vi "log_key_variant.vi"(8 "error in (no error)":errorcluster, 10 "Ctl Refnum":refnum<vi>, 11 "Byte Stream File in":refnum<file>) -> (0 "error out":errorcluster, 3 "Byte Stream File out":refnum<file>)   [LabVIEW 2015]
doc: "Copyright (c) 2018 Frans Korhonen, Institute for Atmospheric and Earth System Research / Physics, Faculty of Science, University of Helsinki, Finland\n\nThis file is part of MeasGUI.\n\nThis Source Code Form is subject to the terms of the Mozilla Public\nLicense, v. 2.0. If a copy of the MPL was not distributed with this\n file, You can obtain one at http://mozilla.org/MPL/2.0/."
panel:
  out "Value":variant
  out "ClassName":string
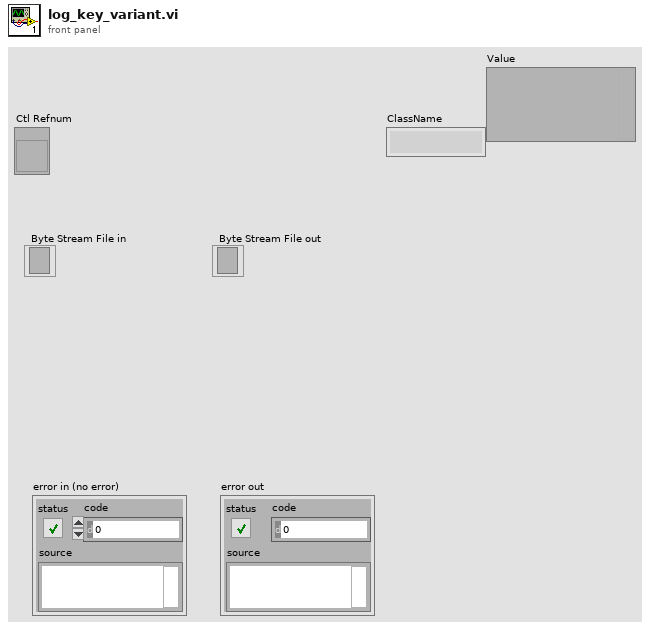
[diagram p1: front panel]
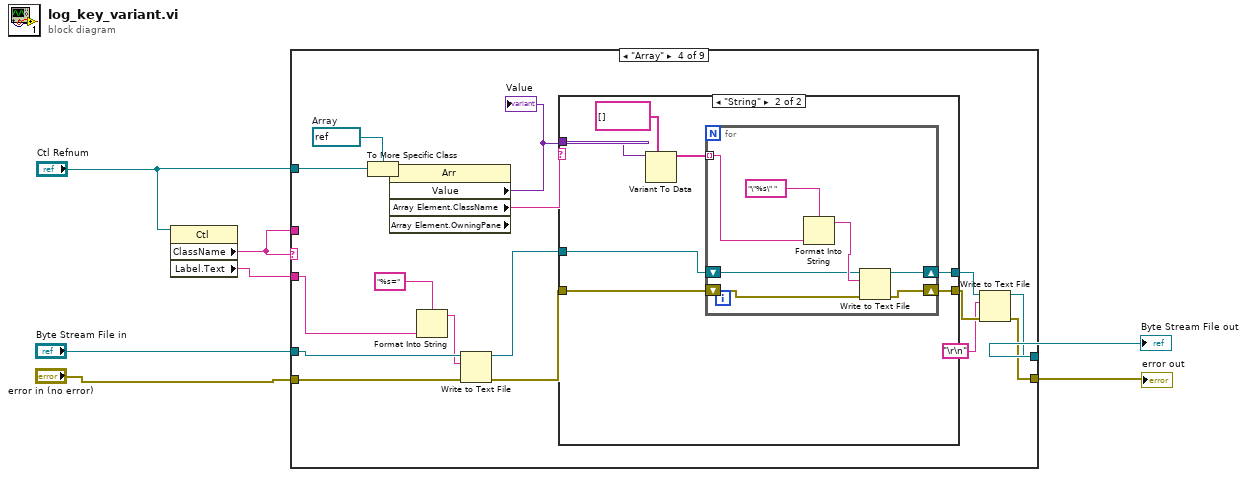
[diagram p0: block diagram]
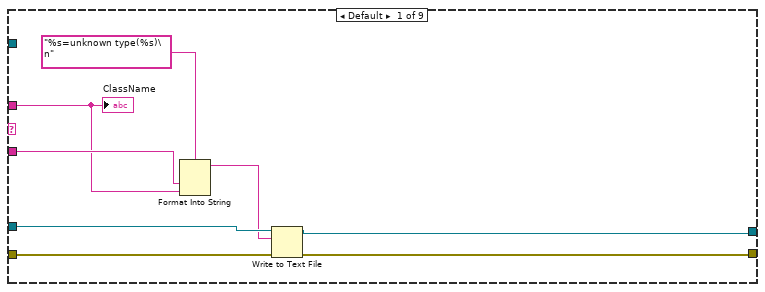
[diagram p2: hidden frame]
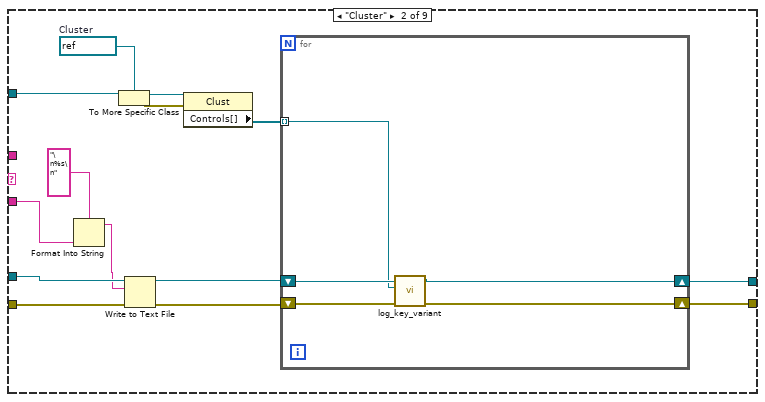
[diagram p3: hidden frame]
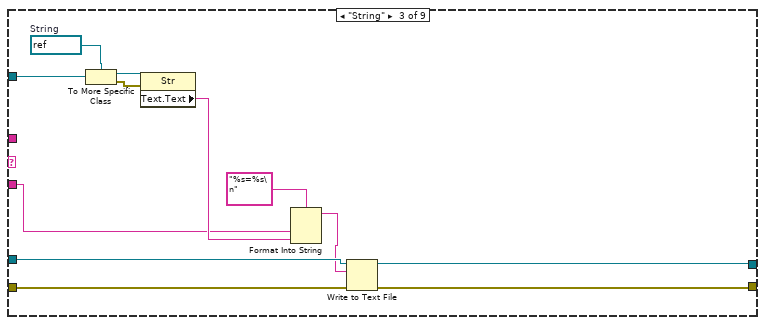
[diagram p4: hidden frame]
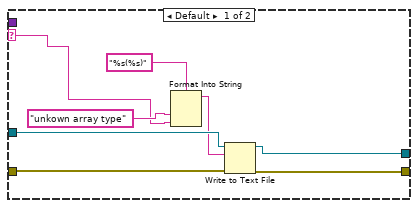
[diagram p5: hidden frame]
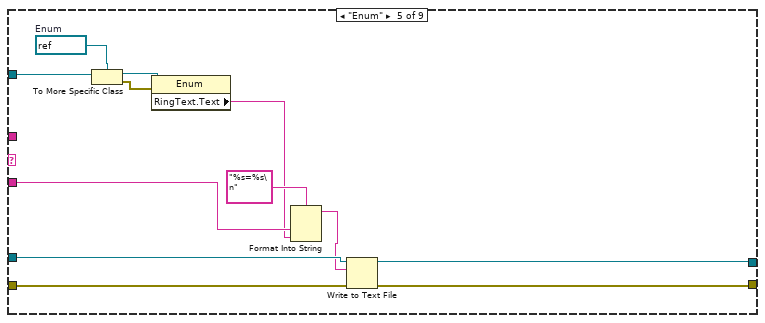
[diagram p6: hidden frame]
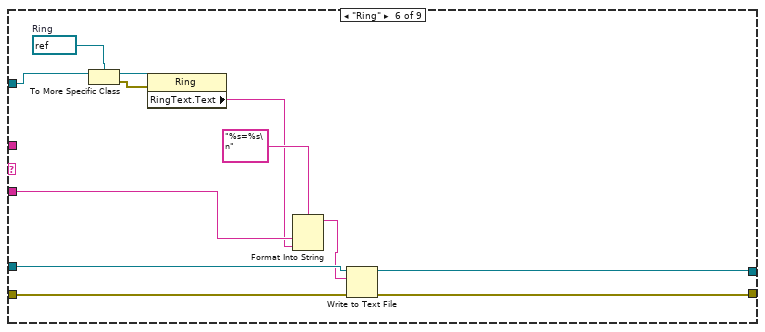
[diagram p7: hidden frame]
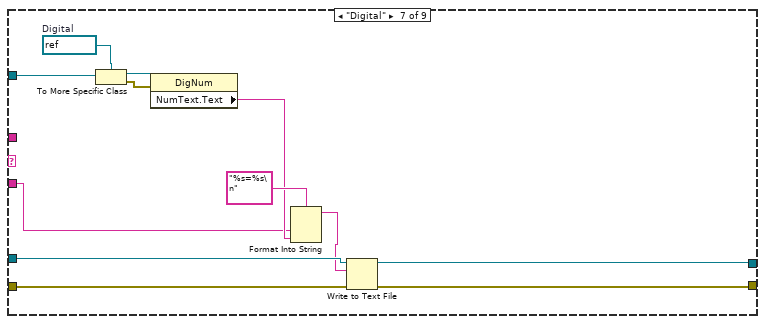
[diagram p8: hidden frame]
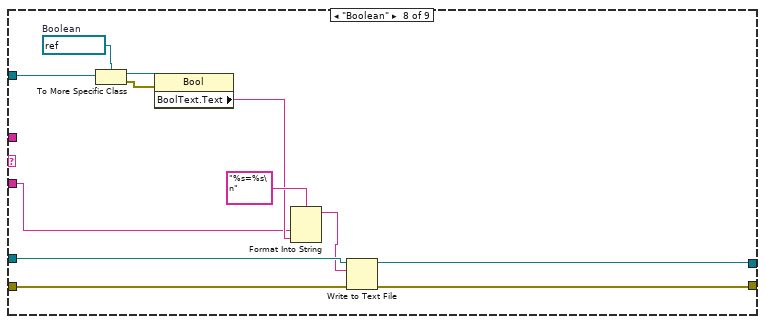
[diagram p9: hidden frame]
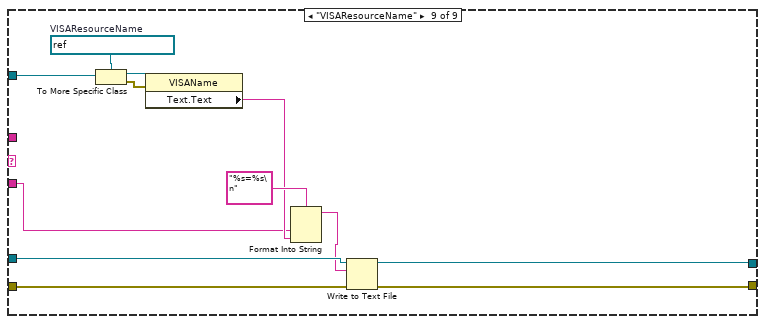
[diagram p10: hidden frame]
diagram:
  n1 = property class="Ctl"(reference="Ctl Refnum") -> ("ClassName"=w7:string, "Label.Text"=w1:string)  [unwired: 1 in, 2 out]
  n2 = case shown="\"Array\"" w7 {
    tunnel: w7 -> [w14 _ _ _ _ _ _ _ _]
    tunnel: "Ctl Refnum" -> [_ w28 w37 w61 w89 w101 w113 w125 w137]
    tunnel: "Byte Stream File in" -> [w12 w24 w46 w50 w98 w110 w122 w134 w146]
    tunnel: "error in (no error)" -> [w11 w23 w43 w51 w95 w107 w119 w131 w143]
    tunnel: [w10 w21 w45 w55 w97 w109 w121 w133 w145] -> w3
    tunnel: [w9 w18 w44 w56 w96 w108 w120 w132 w144] -> w2
    tunnel: w1 -> [w15 w17 w35 w47 w88 w100 w111 w123 w135]
    frame Default {
      n3 = Format Into String(format string="%s=unknown type(%s)\n", w15, w14) -> (resulting string=w8:string)  [unwired: 2 in, 1 out]
      n4 = Write to Text File(file (use dialog)=w12, text=w8, error in=w11) -> (refnum out=w10:refnum<file>, error out=w9:errorcluster)  [unwired: 1 in, 1 out]
      "ClassName" <- w14
    }
    frame "Cluster" {
      w29 = refnum<vi> refnum  # Cluster
      n5 = Format Into String(format string="\n%s\n", w17) -> (resulting string=w16:string)  [unwired: 2 in, 1 out]
      n6 = To More Specific Class(target class=w29, reference=w28) -> (specific class reference=w27:refnum<vi>, error out=w26:errorcluster)  [unwired: 1 in]
      n7 = Write to Text File(file (use dialog)=w24, text=w16, error in=w23) -> (refnum out=w20:refnum<file>, error out=w19:errorcluster)  [unwired: 1 in, 1 out]
      n8 = property class="Clust"(reference=w27, error in=w26) -> ("Controls[]"=w25:refnum<vi>[])  [unwired: 2 out]
      n9 = for {
        tunnel: w25 -> [w30] mode=indexing
        shift-right: [w34] -> w21
        shift-left: w20 -> [w33]
        shift-right: [w31] -> w18
        shift-left: w19 -> [w32]
        n10 = call "log_key_variant.vi"("error in (no error)"=w32, "Ctl Refnum"=w30, "Byte Stream File in"=w33) -> ("error out"=w31:errorcluster, "Byte Stream File out"=w34:refnum<file>)  [unwired: 7 in]
      }
    }
    frame "String" {
      w40 = refnum<vi> refnum  # String
      n11 = To More Specific Class(target class=w40, reference=w37) -> (specific class reference=w38:refnum<vi>, error out=w39:errorcluster)  [unwired: 1 in]
      n12 = property class="Str"(reference=w38, error in=w39) -> ("Text.Text"=w36:string)  [unwired: 2 out]
      n13 = Format Into String(format string="%s=%s\n", w35, w36) -> (resulting string=w42:string)  [unwired: 2 in, 1 out]
      n14 = Write to Text File(file (use dialog)=w46, text=w42, error in=w43) -> (refnum out=w45:refnum<file>, error out=w44:errorcluster)  [unwired: 1 in, 1 out]
    }
    frame "Array" {
      w64 = refnum<vi> refnum  # Array
      n15 = To More Specific Class(target class=w64, reference=w61) -> (specific class reference=w62:refnum<vi>, error out=w63:errorcluster)  [unwired: 1 in]
      n16 = property class="Arr" props=["Value", "Array Element", "ClassName", "Array Element", "OwningPane"](reference=w62, error in=w63) -> ("Value"=w60:variant, "Array Element.ClassName"=w59:string)  [unwired: 3 out]
      "Value" <- w60
      n17 = Format Into String(format string="%s=", w47) -> (resulting string=w49:string)  [unwired: 2 in, 1 out]
      n18 = Write to Text File(file (use dialog)=w50, text=w49, error in=w51) -> (refnum out=w53:refnum<file>, error out=w52:errorcluster)  [unwired: 1 in, 1 out]
      n19 = case shown="\"String\"" w59 {
        selector: w59 -> [w65 _]
        tunnel: w60 -> [_ w79]
        tunnel: w53 -> [w70 w76]
        tunnel: w52 -> [w69 w75]
        tunnel: [w72 w74] -> w58
        tunnel: [w71 w73] -> w57
        frame Default {
          n20 = Format Into String(format string="%s(%s)", "unkown array type" ("text"), w65) -> (resulting string=w66:string)  [unwired: 2 in, 1 out]
          n21 = Write to Text File(file (use dialog)=w70, text=w66, error in=w69) -> (refnum out=w72:refnum<file>, error out=w71:errorcluster)  [unwired: 1 in, 1 out]
        }
        frame "String" {
          n22 = Variant To Data(type=string[] [], Variant=w79) -> (data=w77:string[])  [unwired: 1 in, 1 out]
          n23 = for {
            tunnel: w77 -> [w80] mode=indexing
            shift-right: [w81] -> w74
            shift-left: w76 -> [w84]
            shift-right: [w82] -> w73
            shift-left: w75 -> [w83]
            n24 = Format Into String(format string="\"%s\" ", w80) -> (resulting string=w86:string)  [unwired: 2 in, 1 out]
            n25 = Write to Text File(file (use dialog)=w84, text=w86, error in=w83) -> (refnum out=w81:refnum<file>, error out=w82:errorcluster)  [unwired: 1 in, 1 out]
          }
        }
      }
      n26 = Write to Text File(file (use dialog)=w58, text="\r\n", error in=w57) -> (refnum out=w55:refnum<file>, error out=w56:errorcluster)  [unwired: 1 in, 1 out]
    }
    frame "Enum" {
      w92 = refnum<vi> refnum  # Enum
      n27 = To More Specific Class(target class=w92, reference=w89) -> (specific class reference=w90:refnum<vi>, error out=w91:errorcluster)  [unwired: 1 in]
      n28 = property class="Enum"(reference=w90, error in=w91) -> ("RingText.Text"=w87:string)  [unwired: 2 out]
      n29 = Format Into String(format string="%s=%s\n", w88, w87) -> (resulting string=w94:string)  [unwired: 2 in, 1 out]
      n30 = Write to Text File(file (use dialog)=w98, text=w94, error in=w95) -> (refnum out=w97:refnum<file>, error out=w96:errorcluster)  [unwired: 1 in, 1 out]
    }
    frame "Ring" {
      w104 = refnum<vi> refnum  # Ring
      n31 = To More Specific Class(target class=w104, reference=w101) -> (specific class reference=w102:refnum<vi>, error out=w103:errorcluster)  [unwired: 1 in]
      n32 = property class="Ring"(reference=w102, error in=w103) -> ("RingText.Text"=w99:string)  [unwired: 2 out]
      n33 = Format Into String(format string="%s=%s\n", w100, w99) -> (resulting string=w106:string)  [unwired: 2 in, 1 out]
      n34 = Write to Text File(file (use dialog)=w110, text=w106, error in=w107) -> (refnum out=w109:refnum<file>, error out=w108:errorcluster)  [unwired: 1 in, 1 out]
    }
    frame "Digital" {
      w114 = refnum<vi> refnum  # Digital
      n35 = To More Specific Class(target class=w114, reference=w113) -> (specific class reference=w116:refnum<vi>, error out=w115:errorcluster)  [unwired: 1 in]
      n36 = property class="DigNum"(reference=w116, error in=w115) -> ("NumText.Text"=w112:string)  [unwired: 2 out]
      n37 = Format Into String(format string="%s=%s\n", w111, w112) -> (resulting string=w118:string)  [unwired: 2 in, 1 out]
      n38 = Write to Text File(file (use dialog)=w122, text=w118, error in=w119) -> (refnum out=w121:refnum<file>, error out=w120:errorcluster)  [unwired: 1 in, 1 out]
    }
    frame "Boolean" {
      w126 = refnum<vi> refnum  # Boolean
      n39 = To More Specific Class(target class=w126, reference=w125) -> (specific class reference=w128:refnum<vi>, error out=w127:errorcluster)  [unwired: 1 in]
      n40 = property class="Bool"(reference=w128, error in=w127) -> ("BoolText.Text"=w124:string)  [unwired: 2 out]
      n41 = Format Into String(format string="%s=%s\n", w123, w124) -> (resulting string=w130:string)  [unwired: 2 in, 1 out]
      n42 = Write to Text File(file (use dialog)=w134, text=w130, error in=w131) -> (refnum out=w133:refnum<file>, error out=w132:errorcluster)  [unwired: 1 in, 1 out]
    }
    frame "VISAResourceName" {
      w138 = refnum<vi> refnum  # VISAResourceName
      n43 = To More Specific Class(target class=w138, reference=w137) -> (specific class reference=w140:refnum<vi>, error out=w139:errorcluster)  [unwired: 1 in]
      n44 = property class="VISAName"(reference=w140, error in=w139) -> ("Text.Text"=w136:string)  [unwired: 2 out]
      n45 = Format Into String(format string="%s=%s\n", w135, w136) -> (resulting string=w142:string)  [unwired: 2 in, 1 out]
      n46 = Write to Text File(file (use dialog)=w146, text=w142, error in=w143) -> (refnum out=w145:refnum<file>, error out=w144:errorcluster)  [unwired: 1 in, 1 out]
    }
  }
  "error out" <- w2
  "Byte Stream File out" <- w3
